vi "build error object.vi"(6 "Time Stamp":timestamp, 8 "Error to Process":errorcluster, 9 "Report Error (F)":bool, 10 "Severity (Do Nothing)":T1, 11 "Error Location":refnum<class>) -> (3 "Error object":refnum<class "Error.lvclass">)   [LabVIEW 2020, in "Error Interface.lvlib" / "Error.lvclass"]
uses:
  Error.lvclass
  typedefs/error severity.ctl
  Error.lvclass/Error.ctl
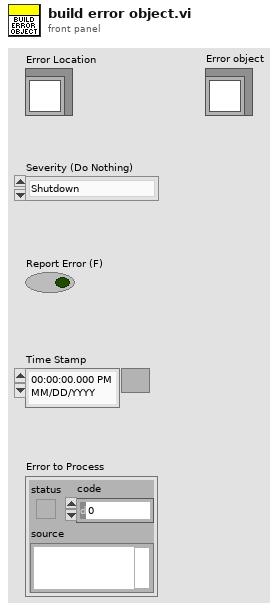
[diagram p1: front panel]
types:
  T1 = typedef "Error Interface.lvlib/Error.lvclass/error severity.ctl" = enum16{"Shutdown", "Restart Calling Actor", "Restart Nested Actor", "Do Nothing"}
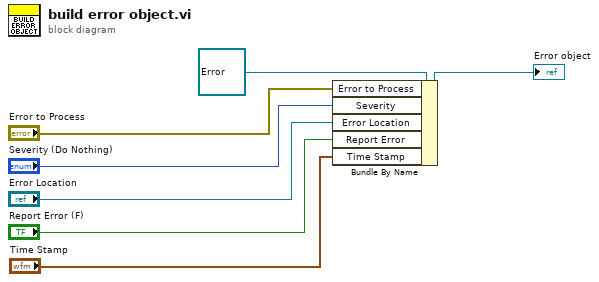
[diagram p0: block diagram]
diagram:
  n1 = Bundle By Name(cluster=refnum<class "Error.lvclass"> refnum ("Error object"), "Error to Process"="Error to Process", "Severity"="Severity (Do Nothing)", "Error Location"="Error Location", "Report Error"="Report Error (F)", "Time Stamp"="Time Stamp") -> (→"Error object":refnum<class "Error.lvclass">)
